vi "Initialization VI.vi"(8 "error in (no error)":errorcluster, 10 "Custom XML":string, 11 "Device Item Ref in":T1 format="%.0x") -> (0 "error out":errorcluster, 3 "Device Item Ref out":T1 format="%.0x")   [LabVIEW 2021, in "gRPC Data Server System Explorer.lvlib"]
uses:
  gRPC Data Server System Explorer.lvlib
  <vilib>/NI VeriStand/Custom Device API/Custom Device Item Ref.ctl
  <vilib>/NI VeriStand/Custom Device API/Custom Device Channel.ctl
  <vilib>/NI VeriStand/Custom Device API/Custom Device Channel Type.ctl
  Shared/Compiled.Settings.ctl
  <vilib>/NI VeriStand/Custom Device API/Custom Device File Dependency.ctl
  <vilib>/NI VeriStand/Custom Device API/Path Specification.ctl
  <vilib>/NI VeriStand/Custom Device API/Path Type.ctl
  <vilib>/NI VeriStand/Custom Device API/Custom Device Supported Target.ctl
  Shared/Constants.vi
  <vilib>/NI VeriStand/Custom Device API/Custom Device API.lvlib
  Shared/gRPC Data Server Shared.lvlib
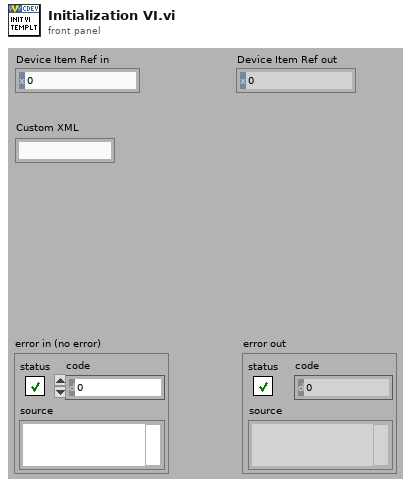
[diagram p1: front panel]
types:
  T1 = typedef "Custom Device API.lvlib/Custom Device Item Ref.ctl" = u64
  T2 = typedef "Custom Device API.lvlib/Custom Device Supported Target.ctl" = enum16{"All", "PharLap", "VxWorks", "Windows", "Linux_32_ARM", "Linux_x64", "PharLap & Windows", "PharLap & VxWorks", "VxWorks & Windows"}
  T3 = typedef "Custom Device API.lvlib/Path Type.ctl" = enum16{"Absolute", "To Base", "To Common Data Dir", "To Application Data Dir"}
  T4 = typedef "Custom Device API.lvlib/Custom Device File Dependency.ctl" = cluster{"Source":T5, "RT Destination":path, "ForceDownload?":bool, "SupportedTarget":T2, "Version":string}
  T5 = typedef "Custom Device API.lvlib/Path Specification.ctl" = cluster{"Path":path, "Type":T3}
  T6 = typedef "gRPC Data Server Shared.lvlib/Compiled.Settings.ctl" = cluster{"Name":string, "Server Address":string, "Async?":bool, "Key File":path, "Cert File":path, "Channel Name":string[], "Initial Value":string[]}
  T7 = typedef "Custom Device API.lvlib/Custom Device Channel.ctl" = cluster{"Type":T8, "Units":string, "Default Value":dbl, "Faultable":bool, "Scalable":bool}
  T8 = typedef "Custom Device API.lvlib/Custom Device Channel Type.ctl" = enum16{"Input", "Output"}
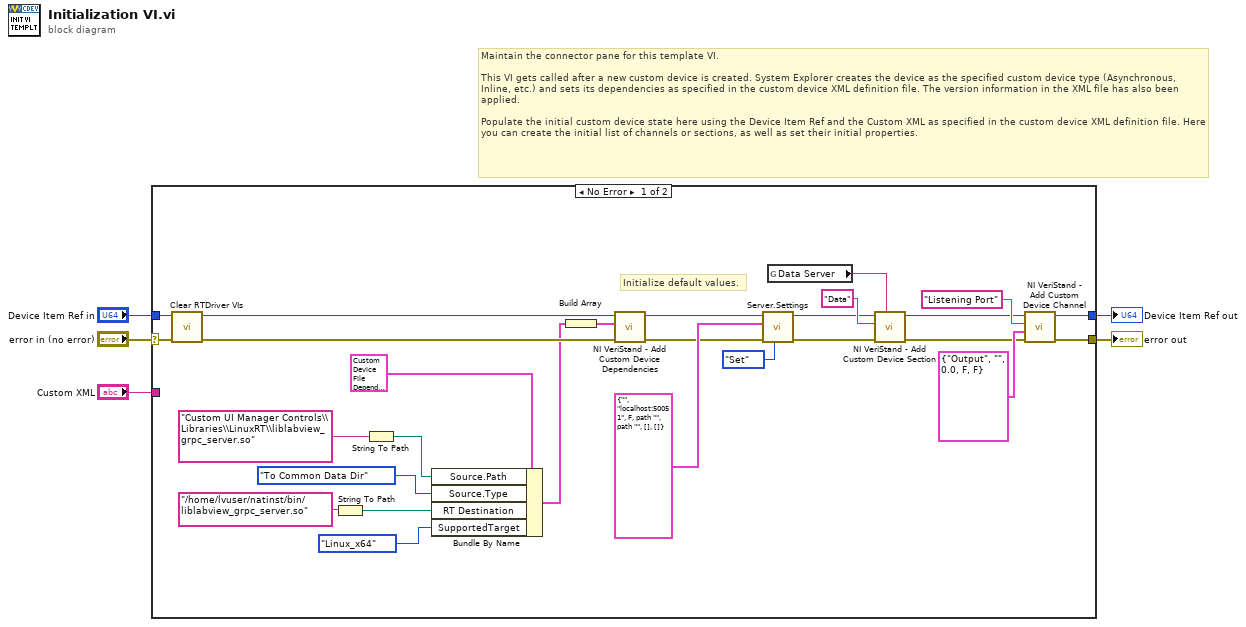
[diagram p0: block diagram]
diagram:
  # "Maintain the connector pane for this template VI.\n\nThis VI gets called after a new custom device is created. System Explorer creates the device as the specified custom device type (Asynchronous, Inline, etc.) and sets its dependencies as specified in the custom device XML definition file. The version information in the XML file has also been applied.\n\nPopulate the initial custom device state here using the Device Item Ref and the Custom XML as specified in the custom device XML definition file. Here you can create the initial list of channels or sections, as well as set their initial properties."
  n1 = case shown="No Error" "error in (no error)" {
    selector: "error in (no error)" -> [w19 w34]
    tunnel: [w27 w34] -> w5
    tunnel: [w28 w33] -> w3
    tunnel: "Device Item Ref in" -> [w20 w33]
    tunnel: "Custom XML" -> [_ _]
    frame No Error {
      # "Initialize default values."
      n2 = call "Clear RTDriver VIs.vi"("error in (no error)"=w19, "Device Item Ref in in"=w20) -> ("error out"=w16:errorcluster, "Device Item Ref out"=w18:T1)  [unwired: 8 in]
      n3 = String To Path(string="/home/lvuser/natinst/bin/liblabview_grpc_server.so") -> (path=w7:path)
      n4 = String To Path(string="Custom UI Manager Controls\\Libraries\\LinuxRT\\liblabview_grpc_server.so") -> (path=w8:path)
      n5 = Bundle By Name(cluster=T4 {"Source"={"Path"=path "", "Type"=enum."Absolute"}, "RT Destination"=path "", "ForceDownload?"=FALSE, "SupportedTarget"=enum."PharLap", "Version"=""} ("Dependency"), "Source.Path"=w8, "Source.Type"=Path_Type."To Common Data Dir", "RT Destination"=w7, "SupportedTarget"=Custom_Device_Supported_Target."Linux_x64") -> (w13:T4)
      n6 = Build Array(w13) -> (w12:T4[])
      n7 = call <vilib>:"NI VeriStand - Add Custom Device Dependencies.vi"("error in (no error)"=w16, "Dependencies"=w12, "Device Ref in"=w18) -> ("error out"=w15:errorcluster, "Device Ref out"=w17:T1)  [unwired: 7 in]
      n8 = call "Server.Settings.vi"("Action"=enum8{"Get", "Set"}."Set", "error in (no error)"=w15, "Settings In"=T6 {"Name"="", "Server Address"="localhost:50051", "Async?"=FALSE, "Key File"=path "", "Cert File"=path "", "Channel Name"=[], "Initial Value"=[]} ("Client Settings In"), "Parent Ref in"=w17) -> ("error out"=w21:errorcluster, "Item Ref out"=w22:T1)  [unwired: 5 in, 1 out]
      n9 = global read "Constants.vi" "Data Server"() -> (w25:string)
      n10 = call <vilib>:"NI VeriStand - Add Custom Device Section.vi"("GUID (Default Section)"=w25, "error in (no error)"=w21, "Section Name"="Data", "Parent Ref in"=w22) -> ("error out"=w29:errorcluster, "Parent Ref out"=w30:T1)  [unwired: 4 in, 2 out]
      n11 = call <vilib>:"NI VeriStand - Add Custom Device Channel.vi"("error in (no error)"=w29, "Channel"=T7 {"Type"=enum."Output", "Units"="", "Default Value"=0.0, "Faultable"=FALSE, "Scalable"=FALSE}, "Channel Name"="Listening Port", "Parent Ref in"=w30) -> ("error out"=w27:errorcluster, "Parent Ref out"=w28:T1)  [unwired: 4 in, 2 out]
    }
    frame Error {
    }
  }
  "error out" <- w5
  "Device Item Ref out" <- w3
